vi "CheckParamerter.vi"(8 "error in (no error)":errorcluster, 11 "Array":i32[](array[numeric])) -> (0 "error out":errorcluster)   [LabVIEW 2013]
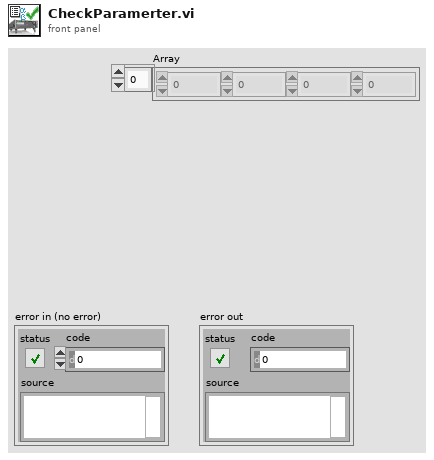
[diagram p1: front panel]
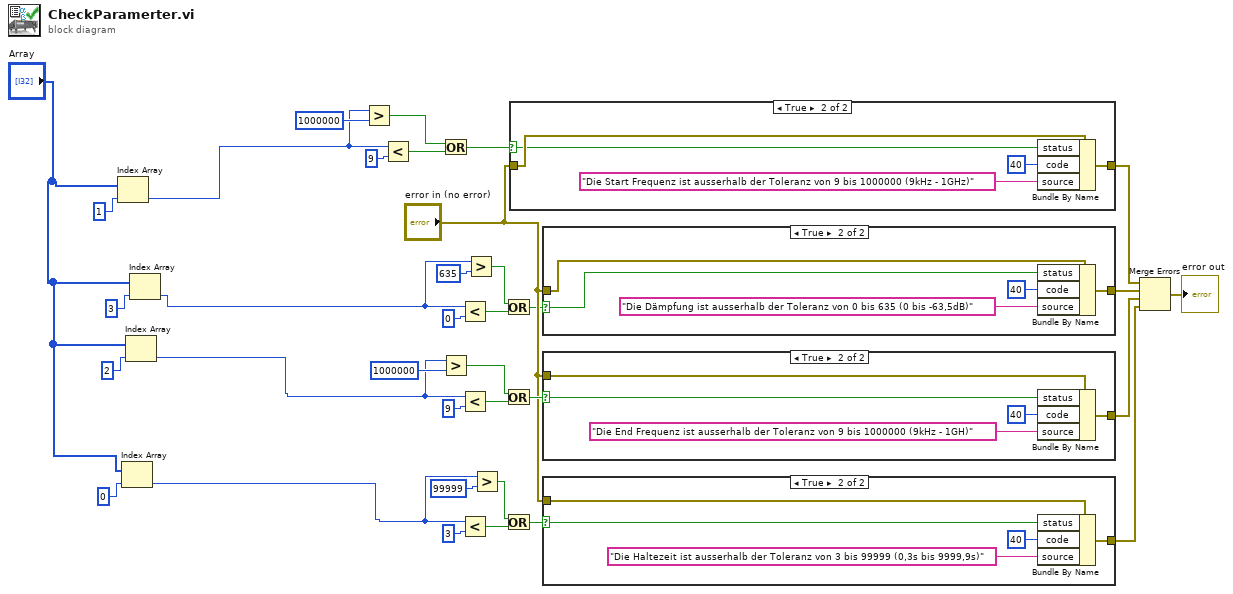
[diagram p0: block diagram]
diagram:
  n1 = Index Array(array="Array", index=1) -> (element=w4:i32)
  n2 = Index Array(array="Array", index=0) -> (element=w1:i32)
  n3 = Index Array(array="Array", index=2) -> (element=w2:i32)
  n4 = Index Array(array="Array", index=3) -> (element=w3:i32)
  n5 = Greater?(x=w4, y=u32 1000000) -> (0:w12:bool)
  n6 = Less?(x=w4, y=u32 9) -> (x < y?=w11:bool)
  n7 = Or(x=w12, y=w11) -> (x .or. y?=w26:bool)
  n8 = Greater?(x=w2, y=u32 1000000) -> (0:w20:bool)
  n9 = Less?(x=w3, y=u32 0) -> (x < y?=w15:bool)
  n10 = Less?(x=w2, y=u32 9) -> (x < y?=w19:bool)
  n11 = Less?(x=w1, y=u32 3) -> (x < y?=w23:bool)
  n12 = Greater?(x=w3, y=u32 635) -> (0:w16:bool)
  n13 = Greater?(x=w1, y=u32 99999) -> (0:w24:bool)
  n14 = Or(x=w16, y=w15) -> (x .or. y?=w27:bool)
  n15 = Or(x=w20, y=w19) -> (x .or. y?=w30:bool)
  n16 = Or(x=w24, y=w23) -> (x .or. y?=w29:bool)
  n17 = case shown="True" w26 {
    selector: w26 -> [_ w40]
    tunnel: "error in (no error)" -> [w36 w41]
    tunnel: [w36 w37] -> w31
    frame False {
    }
    frame True {
      n18 = Bundle By Name(cluster=w41, "status"=w40, "code"=40, "source"="Die Start Frequenz ist ausserhalb der Toleranz von 9 bis 1000000 (9kHz - 1GHz)") -> (w37:errorcluster)
    }
  }
  n19 = case shown="True" w27 {
    selector: w27 -> [_ w46]
    tunnel: "error in (no error)" -> [w42 w47]
    tunnel: [w42 w43] -> w32
    frame False {
    }
    frame True {
      n20 = Bundle By Name(cluster=w47, "status"=w46, "code"=40, "source"="Die Dämpfung ist ausserhalb der Toleranz von 0 bis 635 (0 bis -63,5dB)") -> (w43:errorcluster)
    }
  }
  n21 = case shown="True" w30 {
    selector: w30 -> [_ w52]
    tunnel: "error in (no error)" -> [w48 w53]
    tunnel: [w48 w49] -> w33
    frame False {
    }
    frame True {
      n22 = Bundle By Name(cluster=w53, "status"=w52, "code"=40, "source"="Die End Frequenz ist ausserhalb der Toleranz von 9 bis 1000000 (9kHz - 1GH)") -> (w49:errorcluster)
    }
  }
  n23 = case shown="True" w29 {
    selector: w29 -> [_ w59]
    tunnel: [w54 w56] -> w34
    tunnel: "error in (no error)" -> [w54 w55]
    frame False {
    }
    frame True {
      n24 = Bundle By Name(cluster=w55, "status"=w59, "code"=40, "source"="Die Haltezeit ist ausserhalb der Toleranz von 3 bis 99999 (0,3s bis 9999,9s)") -> (w56:errorcluster)
    }
  }
  n25 = Merge Errors(w31, w32, w33, w34) -> (→"error out":errorcluster)
